vi "State vector.vi"(9 "Final state? (T)":bool=TRUE, 11 "Circuit cluster":T1) -> (3 "State vector":cdb[](array[numeric]) format="%#_3g")   [LabVIEW 2016]
uses:
  TypeDefs/Circuit Cluster.ctl
  Classes/GateAbst/GateAbst.lvclass
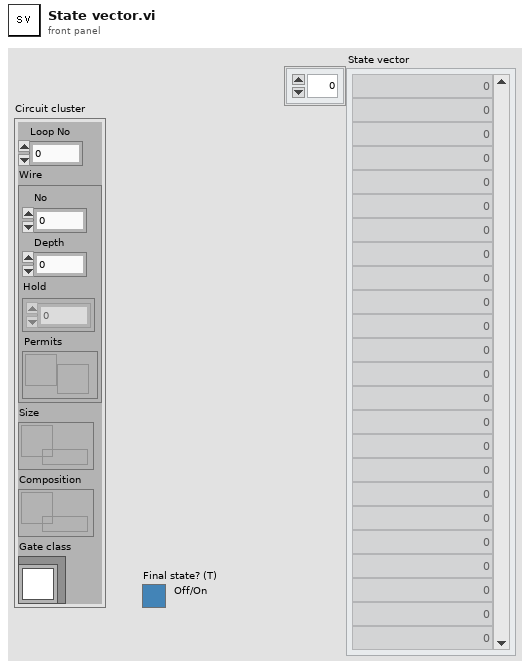
[diagram p1: front panel]
types:
  T1 = typedef "Circuit Cluster.ctl" = cluster{"Loop No":i32, "Wire":cluster{"No":i32, "Depth":i32, "Hold":i32[][], "Permits":refnum<notifier>}, "Size":refnum<queue>, "Composition":refnum<queue>, "Gate class":refnum<class "GateAbst.lvclass">}
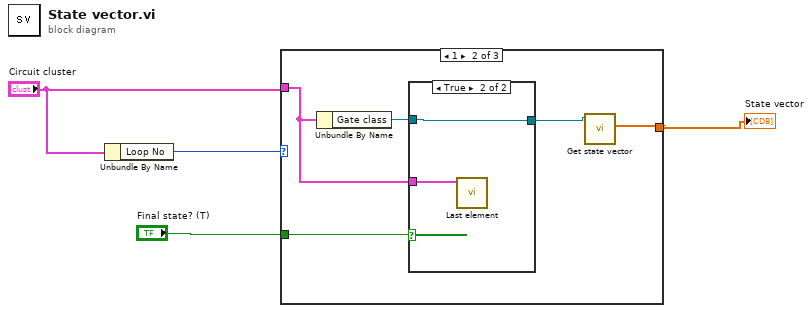
[diagram p0: block diagram]
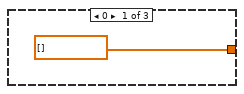
[diagram p2: hidden frame]
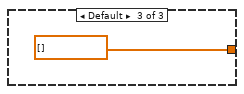
[diagram p4: hidden frame]
diagram:
  n1 = Unbundle By Name("Circuit cluster") -> ("Loop No"=w1:i32)
  n2 = case shown="1" w1 {
    tunnel: "Circuit cluster" -> [_ w8 _]
    tunnel: [cdb[] [] ("State vector") w10 cdb[] [] ("State vector")] -> w4
    tunnel: "Final state? (T)" -> [_ w9 _]
    frame 0 {
    }
    frame 1 {
      n3 = Unbundle By Name(w8) -> ("Gate class"=w7:refnum<class "GateAbst.lvclass">)
      n4 = case shown="True" w9 {
        tunnel: w8 -> [_ w13]
        tunnel: w7 -> [w11 w12]
        tunnel: [w11 w12] -> w6
        frame False {
        }
        frame True {
          n5 = call "Last element.vi"("Circuit cluster"=w13) -> ()  [unwired: 10 in, 1 out]
        }
      }
      n6 = call-dynamic "Get state vector.vi"("GateAbst in"=w6) -> ("State vector"=w10:cdb[])  [unwired: 8 in, 2 out]
    }
    frame Default {
    }
  }
  "State vector" <- w4
